vi "test-single-adam-functions.vi"() -> ()   [LabVIEW 2020]
uses:
  <vilib>/Instr/_visa.llb/VISA Configure Serial Port (Instr).vi
panel:
  out "acknowledge char":string
  out "success?":bool
  in  "send command":bool
  out "Command Out":string
  in  "Stop":bool
  in  "Output State":bool
  in  "DO Number":u8
  out "error IO":errorcluster
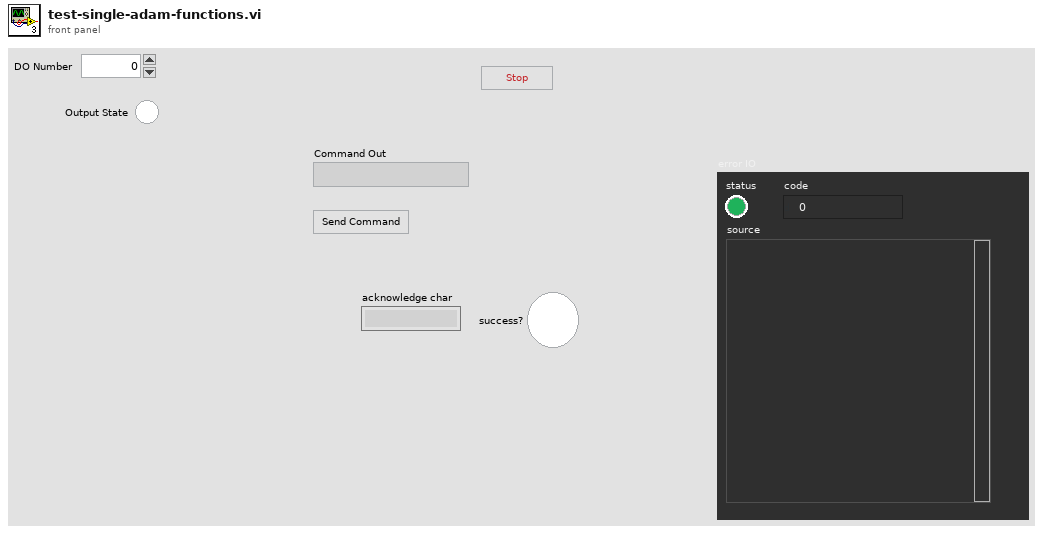
[diagram p1: front panel]
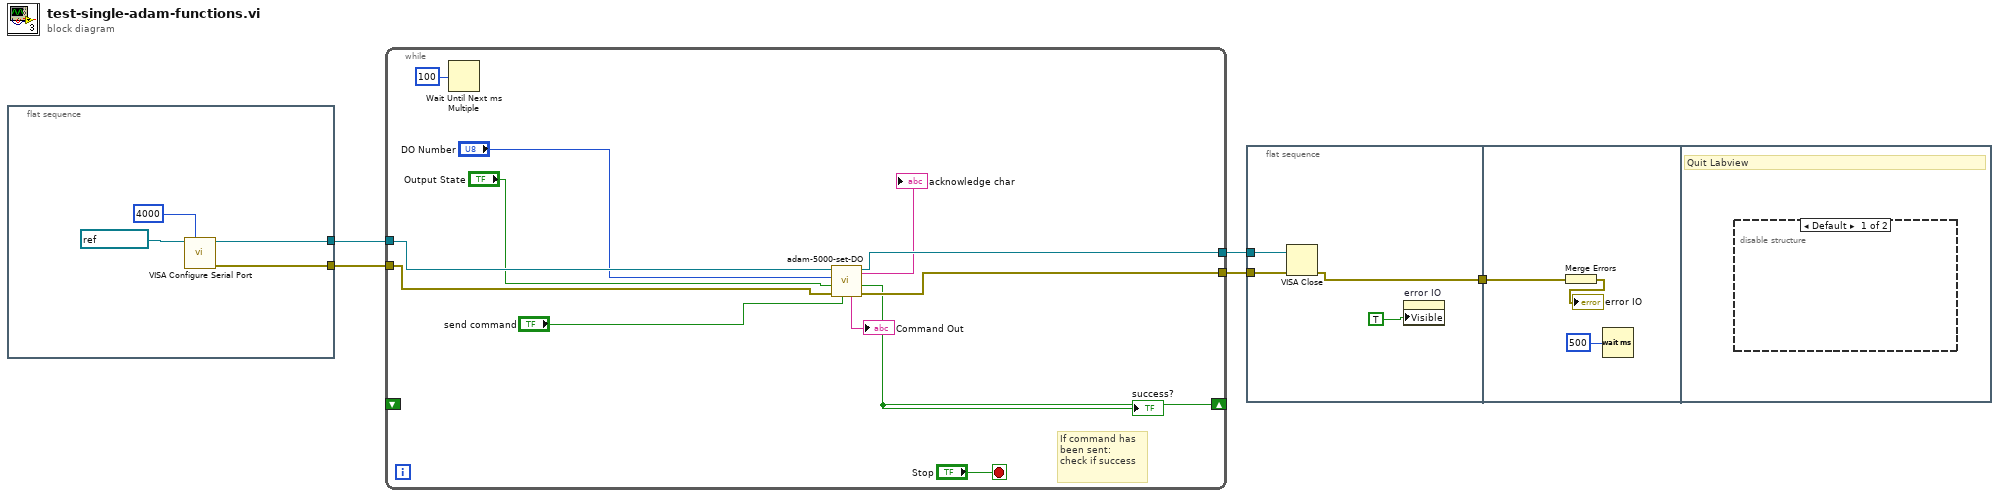
[diagram p0: block diagram]
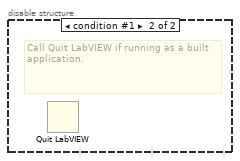
[diagram p2: hidden frame]
diagram:
  n1 = flat-sequence {
    tunnel: [w7] -> w5
    tunnel: [w6] -> w4
    frame #0 {
      n2 = call-poly "VISA Configure Serial Port"("VISA resource name"=refnum<visa-resource-name> "COM10", "timeout (10sec)"=u32 4000) -> ("VISA resource name out"=w7:refnum<visa-resource-name>, "error out"=w6:errorcluster)  [unwired: 12 in]
    }
  }
  n3 = while {
    tunnel: w5 -> [w21]
    tunnel: w4 -> [w20]
    tunnel: [w17] -> w2
    tunnel: [w16] -> w1
    shift-right: [w11] -> _
    shift-left: _ -> [_]
    stop <- "Stop" stop-if-true
    # "If command has\nbeen sent:\ncheck if success"
    n4 = Wait Until Next ms Multiple(millisecond multiple=u32 100) -> ()  [unwired: 1 out]
    n5 = call "adam-5000-set-DO.vi"("send command"="send command", "error in (no error)"=w20, "Output State"="Output State", "DO Number"="DO Number", "VISA Refnum in"=w21) -> ("error out"=w17:errorcluster, "success?"=w11:bool, "VISA Refnum out"=w16:refnum<visa-resource-name>, "Command Used"=→"Command Out":string, "acknowledge char"=→"acknowledge char":string)  [unwired: 1 in, 1 out]
    "success?" <- w11
  }
  n6 = flat-sequence {
    tunnel: w1 -> [w23]
    tunnel: w2 -> [w24]
    tunnel: [w22] -> w3
    tunnel: w3 -> [w26]
    frame #0 {
      n7 = VISA Close(VISA resource name=w23, error in (no error)=w24) -> (error out=w22:errorcluster)
      n8 = property on="error IO" class="Clust (strict)"("Visible"=TRUE) -> ()  [unwired: 2 in, 2 out]
    }
    frame #1 {
      n9 = Merge Errors(w26) -> (→"error IO":errorcluster)
      n10 = Wait (ms)(milliseconds to wait=u32 500) -> ()  [unwired: 1 out]
    }
    frame #2 {
      # "Quit Labview"
      n11 = disable-structure "Conditional Disable Structure" shown="Default" {
        frame condition #0 (active) {
        }
        frame condition #1 {
          # "Call Quit LabVIEW if running as a built application."
          n12 = Quit LabVIEW() -> ()  [unwired: 1 in]
        }
      }
    }
  }
